vi "Initialise.vi"() -> ()   [LabVIEW 2017]
uses:
  TypeDefs/Position-Info-TD.ctl
  Globals/Trav-Positon-Info.vi
panel:
  in  "Position Info":T1
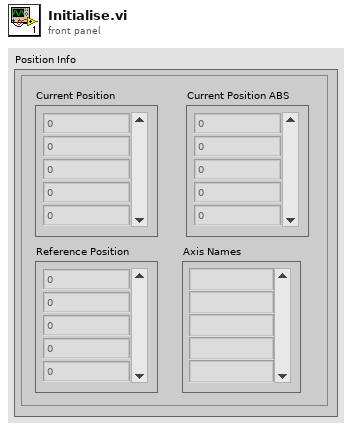
[diagram p1: front panel]
types:
  T1 = typedef "Position-Info-TD.ctl" = cluster{"Current Position ABS":dbl[], "Current Position":dbl[], "Reference Position":dbl[], "Axis Names":string[]}
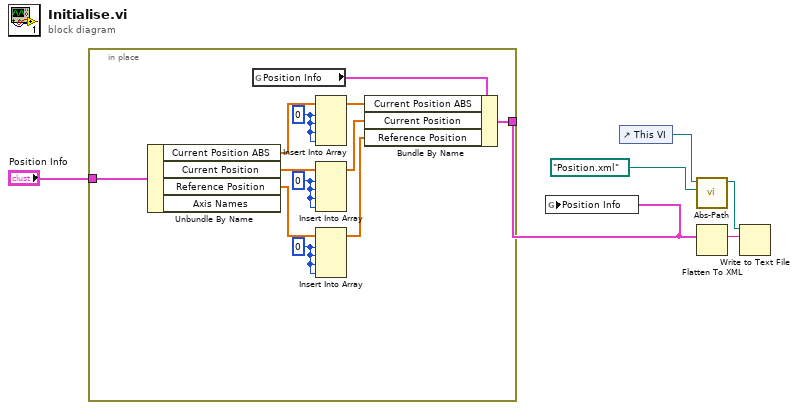
[diagram p0: block diagram]
diagram:
  n1 = in-place {
    in-place-border: "Position Info" -> [w18]
    in-place-border: [w16] -> w1
    w11 = 0 ("index")
    w12 = 0 ("index")
    w13 = 0 ("index")
    n2 = Unbundle By Name(w18) -> ("Current Position ABS"=w17:dbl[], "Current Position"=w10:dbl[], "Reference Position"=w9:dbl[])  [unwired: 1 out]
    n3 = global read "Trav-Positon-Info.vi" "Position Info"() -> (w15:T1)
    n4 = Insert Into Array(array=w17, index=w13, new element #1=w13, new element #2=w13, new element #3=w13) -> (w14:dbl[])
    n5 = Insert Into Array(array=w10, index=w12, new element #1=w12, new element #2=w12, new element #3=w12) -> (w7:dbl[])
    n6 = Insert Into Array(array=w9, index=w11, new element #1=w11, new element #2=w11, new element #3=w11) -> (w8:dbl[])
    n7 = Bundle By Name(cluster=w15, "Current Position ABS"=w14, "Current Position"=w7, "Reference Position"=w8) -> (w16:T1)
  }
  n8 = global write "Trav-Positon-Info.vi" "Position Info"(w1) -> ()
  n9 = control-ref of="This VI"() -> (w5:refnum<vi>)
  n10 = call "Abs-Path.vi"("filename"=path "Position.xml" ("file (use dialog)"), "Vi in path"=w5) -> ("Full path"=w6:path)  [unwired: 9 in]
  n11 = Flatten To XML(anything=w1) -> (xml string=w3:string)
  n12 = Write to Text File(file (use dialog)=w6, text=w3) -> ()  [unwired: 2 in, 3 out]
